vi "FTW-TransferClient-Callback-ProgressUpload.vi"(4 "Initial Parameters":T1 {"Initial Time" format="%.4psec"}, 5 "Event Data":cluster{"sender":refnum<k24>, "e":refnum<k24>}, 6 "Control Ref":refnum<k24>, 7 "Event Common Data":T2) -> ()   [LabVIEW 2015]
uses:
  FTW-TransferClient-TransferProgress.ctl
panel:
  # "Inputs"
  # "Outputs"
  # "No Outputs - this VI\nis fire and forget"
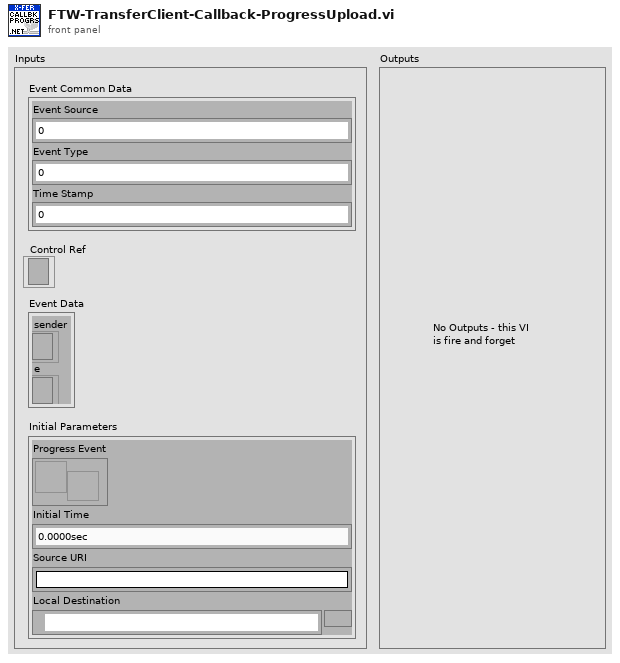
[diagram p1: front panel]
types:
  T1 = cluster{"Progress Event":refnum<user-event>, "Initial Time":dbl, "Source URI":string, "Local Destination":path}
  T2 = cluster{"Event Source":i32, "Event Type":u32, "Time Stamp":u32}
  T3 = typedef "FTW-TransferClient-TransferProgress.ctl" = cluster{"Remote URI":string, "Local Filepath":path, "Total Bytes":i64, "Transferred Bytes":i64, "Percent Complete":dbl, "Current Rate":dbl, "Time Elapsed":dbl, "Estimated Time Remaining":dbl}
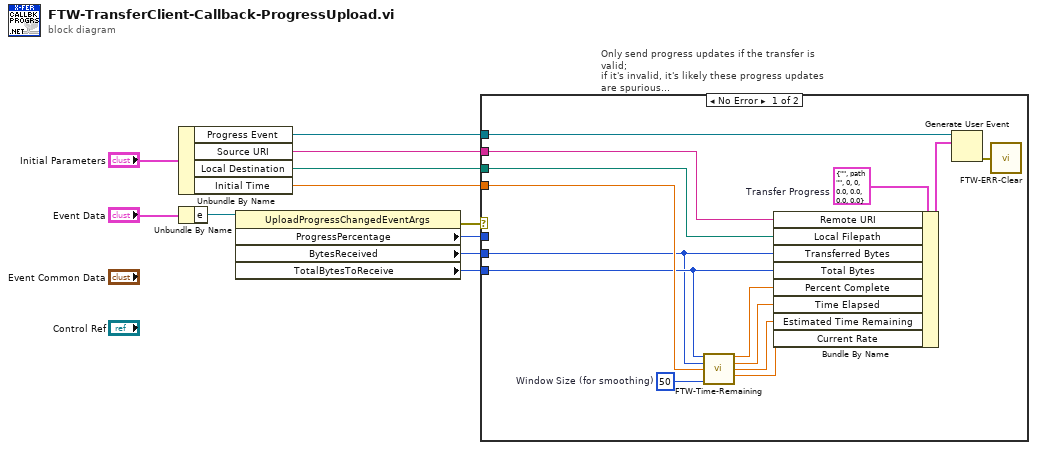
[diagram p0: block diagram]
diagram:
  n1 = Unbundle By Name("Initial Parameters") -> ("Progress Event"=w4:refnum<user-event>, "Source URI"=w11:string, "Local Destination"=w10:path, "Initial Time"=w3:dbl)
  n2 = Unbundle By Name("Event Data") -> ("e"=w5:refnum<k24>)
  n3 = property class="UploadProgressChangedEventArgs"(reference=w5) -> (error out=w6:errorcluster, "ProgressPercentage"=w7:i32, "BytesReceived"=w9:i64, "TotalBytesToReceive"=w8:i64)  [unwired: 1 in, 1 out]
  n4 = case "Only send progress updates if the transfer is valid;\nif it's invalid, it's likely these progress updates are spurious\nattempts to contact the server (anecdotally)" shown="No Error" w6 {
    tunnel: w3 -> [w16 _]
    tunnel: w11 -> [w15 _]
    tunnel: w10 -> [w14 _]
    tunnel: w9 -> [w12 _]
    tunnel: w8 -> [w13 _]
    tunnel: w7 -> [_ _]
    tunnel: w4 -> [w17 _]
    frame No Error {
      w23 = 50  # Window Size (for smoothing)
      w20 = T3 {"Remote URI"="", "Local Filepath"=path "", "Total Bytes"=0, "Transferred Bytes"=0, "Percent Complete"=0.0, "Current Rate"=0.0, "Time Elapsed"=0.0, "Estimated Time Remaining"=0.0}  # Transfer Progress
      n5 = call "FTW-Time-Remaining.vi"("Total Work Units"=w13, "Work Units Complete"=w12, "Initial Timer Value"=w16, "Window Size (for smoothing)"=w23) -> ("Fraction Done [0.0,1.0]"=w22:dbl, "Elapsed Time"=w21:dbl, "Estimated Time Remaining"=w25:dbl, "Current Rate (work/sec)"=w24:dbl)  [unwired: 7 in, 1 out]
      n6 = Bundle By Name(cluster=w20, "Remote URI"=w15, "Local Filepath"=w14, "Transferred Bytes"=w12, "Total Bytes"=w13, "Percent Complete"=w22, "Time Elapsed"=w21, "Estimated Time Remaining"=w25, "Current Rate"=w24) -> (w19:T3)
      n7 = Generate User Event(user event=w17, event data cluster=w19) -> (error out=w18:errorcluster)  [unwired: 2 in, 1 out]
      n8 = call "FTW-ERR-Clear.vi"("error to snuff"=w18) -> ()  [unwired: 1 out]
    }
    frame Error {
    }
  }
